vi "TC_error.vi"() -> ()   [LabVIEW 2014]
panel:
  in  "TC 1 In":dbl
  out "TC 1 Out 2":dbl
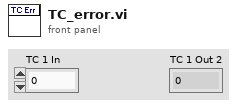
[diagram p1: front panel]
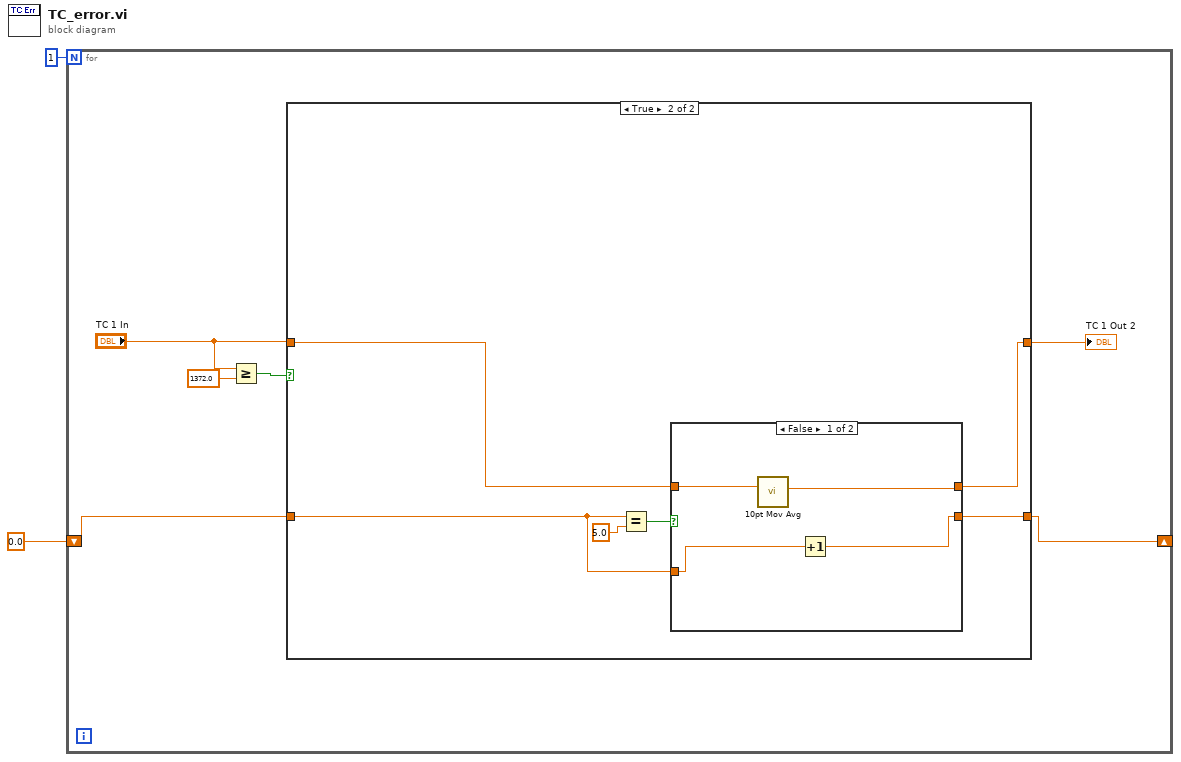
[diagram p0: block diagram]
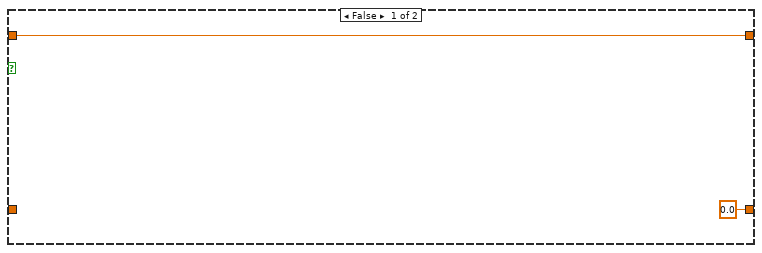
[diagram p2: hidden frame]
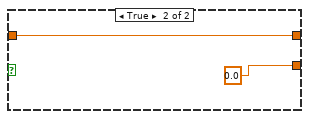
[diagram p3: hidden frame]
diagram:
  n1 = for {
    N: 1 -> [_]
    shift-right: [w6] -> _
    shift-left: 0.0 ("y") -> [w7]
    n2 = Greater Or Equal?(x="TC 1 In", y=1372.0) -> (x >= y?=w5:bool)
    n3 = case shown="True" w5 {
      tunnel: "TC 1 In" -> [w10 w14]
      tunnel: [w10 w13] -> w8
      tunnel: w7 -> [_ w12]
      tunnel: [0.0 ("y") w11] -> w6
      frame False {
      }
      frame True {
        n4 = Equal?(x=w12, y=5.0) -> (x = y?=w16:bool)
        n5 = case shown="False" w16 {
          tunnel: w14 -> [w18 w22]
          tunnel: [w17 w22] -> w13
          tunnel: w12 -> [w20 _]
          tunnel: [w19 0.0 ("y")] -> w11
          frame False {
            n6 = call "10pt Mov Avg.vi"("Value in"=w18) -> ("Value out"=w17:dbl)  [unwired: 10 in]
            n7 = Increment(x=w20) -> (x+1=w19:dbl)
          }
          frame True {
          }
        }
      }
    }
    "TC 1 Out 2" <- w8
  }
